vi "parseBooleanFromLine.vi"(8 "error in (no error)":errorcluster, 9 "engineeringStatus":string, 10 "line":u32, 11 "DomeCommunicator in":refnum<class "DomeCommunicator.lvclass">) -> (0 "error out":errorcluster, 2 "value":bool, 3 "DomeCommunicator out":refnum<class "DomeCommunicator.lvclass">)   [LabVIEW 2016, in "DomeCommunicator.lvclass"]
uses:
  DomeCommunicator.lvclass
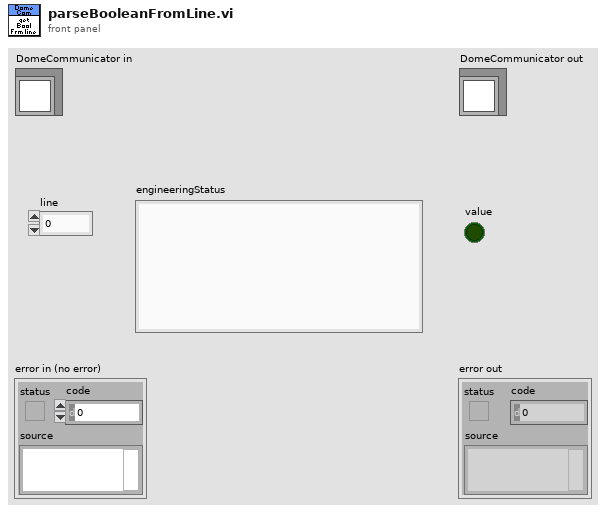
[diagram p1: front panel]
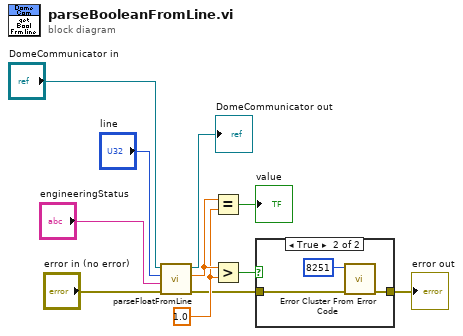
[diagram p0: block diagram]
diagram:
  w4 = sgl 1.0 ("y")
  n1 = call "parseFloatFromLine.vi"("error in (no error)"="error in (no error)", "engineeringStatus"="engineeringStatus", "line"="line", "DomeCommunicator in"="DomeCommunicator in") -> ("error out"=w2:errorcluster, "value"=w5:sgl, "DomeCommunicator out"=→"DomeCommunicator out":refnum<class "DomeCommunicator.lvclass">)  [unwired: 5 in]
  n2 = Equal?(x=w5, y=w4) -> (x = y?=→"value":bool)
  n3 = Greater?(x=w5, y=w4) -> (0:w3:bool)
  n4 = case shown="True" w3 {
    tunnel: w2 -> [w12 w14]
    tunnel: [w12 w15] -> w1
    frame False {
    }
    frame True {
      n5 = call <vilib>:"Error Cluster From Error Code.vi"("error in (no error)"=w14, "error code (0)"=8251) -> ("error out"=w15:errorcluster)  [unwired: 7 in]
    }
  }
  "error out" <- w1
